vi "Set Framed Sensor Path.vi"(8 "error in (no error)":errorcluster, 10 "Framed Sensor Path":path, 11 "Edit Sensor Model in":refnum<class "Edit Sensor Model.lvclass">) -> (0 "error out":errorcluster, 3 "Edit Sensor Model out":refnum<class "Edit Sensor Model.lvclass">)   [LabVIEW 2013, in "Edit Sensor Model.lvlib" / "Edit Sensor Model.lvclass"]
uses:
  Edit Sensor Model.lvclass
  Edit Sensor Model.lvclass/Edit Sensor Model.ctl
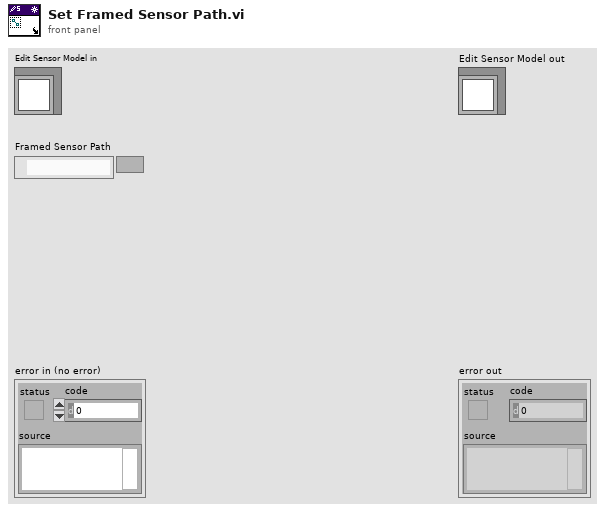
[diagram p1: front panel]
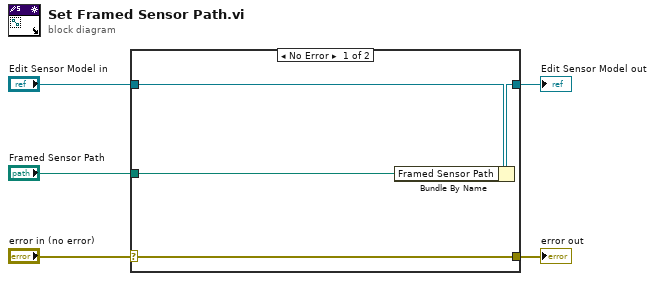
[diagram p0: block diagram]
diagram:
  n1 = case shown="No Error" "error in (no error)" {
    selector: "error in (no error)" -> [w9 w10]
    tunnel: [w9 w10] -> w4
    tunnel: [w7 w11] -> w2
    tunnel: "Edit Sensor Model in" -> [w8 w11]
    tunnel: "Framed Sensor Path" -> [w6 _]
    frame No Error {
      n2 = Bundle By Name(cluster=w8, "Framed Sensor Path"=w6) -> (w7:refnum<class "Edit Sensor Model.lvclass">)
    }
    frame Error {
    }
  }
  "error out" <- w4
  "Edit Sensor Model out" <- w2
